vi "PAM Open TCP Connections.vi"(0 "icListen #":i32=1) -> (1 "TCP IDs":T1, 2 "Error Out":errorcluster)   [LabVIEW 2020]
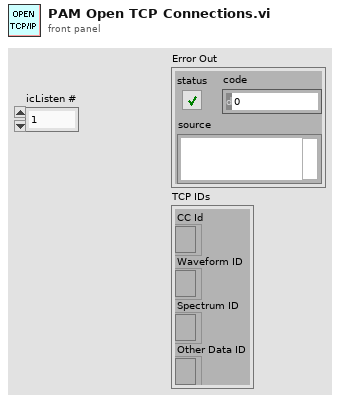
[diagram p1: front panel]
types:
  T1 = cluster{"CC Id":refnum<k5>, "Waveform ID":refnum<k5>, "Spectrum ID":refnum<k5>, "Other Data ID":refnum<k5>}
  T2 = cluster{"connection ID":refnum<k5>, "connection ID":refnum<k5>, "connection ID":refnum<k5>, "connection ID":refnum<k5>}
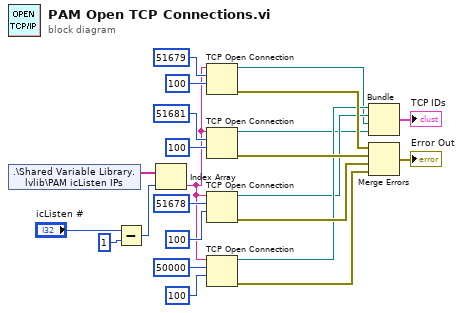
[diagram p0: block diagram]
diagram:
  n1 = shared-variable ".\\Shared Variable Library.lvlib\\PAM icListen IPs"() -> (w13:string[])  [unwired: 1 in, 1 out]
  n2 = Subtract(x="icListen #", y=1) -> (x-y=w1:i32)
  n3 = Index Array(array=w13, index=w1) -> (element=w4:string)
  n4 = TCP Open Connection(address=w4, remote port or service name=u16 51679, timeout ms (60000)=100) -> (connection ID=w16:refnum<k5>, error out=w23:errorcluster)  [unwired: 2 in]
  n5 = TCP Open Connection(address=w4, remote port or service name=u16 51681, timeout ms (60000)=100) -> (connection ID=w15:refnum<k5>, error out=w22:errorcluster)  [unwired: 2 in]
  n6 = TCP Open Connection(address=w4, remote port or service name=u16 51678, timeout ms (60000)=100) -> (connection ID=w17:refnum<k5>, error out=w21:errorcluster)  [unwired: 2 in]
  n7 = TCP Open Connection(address=w4, remote port or service name=u16 50000, timeout ms (60000)=100) -> (connection ID=w18:refnum<k5>, error out=w20:errorcluster)  [unwired: 2 in]
  n8 = Bundle("connection ID"=w18, "connection ID"=w17, "connection ID"=w16, "connection ID"=w15) -> (→"TCP IDs":T2)  [unwired: 1 in]
  n9 = Merge Errors(w23, w22, w21, w20) -> (→"Error Out":errorcluster)
